vi "SA Cond - t0; Merge 2 wForms.vi"(1 "Waveform IN 2":waveform(dbl), 3 "Waveform IN 1":waveform(dbl)) -> (17 "Merged Waveform":waveform(dbl))   [LabVIEW 2022 SP3, in "GSwFormDSP.lvclass"]
uses:
  GSwFormDSP.lvclass
  Generic Utilities_class/Generic Utilities.lvclass
panel:
  out "t0 IN 1 + duration":i64
  out "t0 IN 2":i64
  out "t0 IN 1 + Duration":ext format="%.16f"
  out "t0 IN 2":ext format="%.16f"
  out "t0 IN 1":ext format="%#_24g"
  out "Duration":ext format="%#_24g"
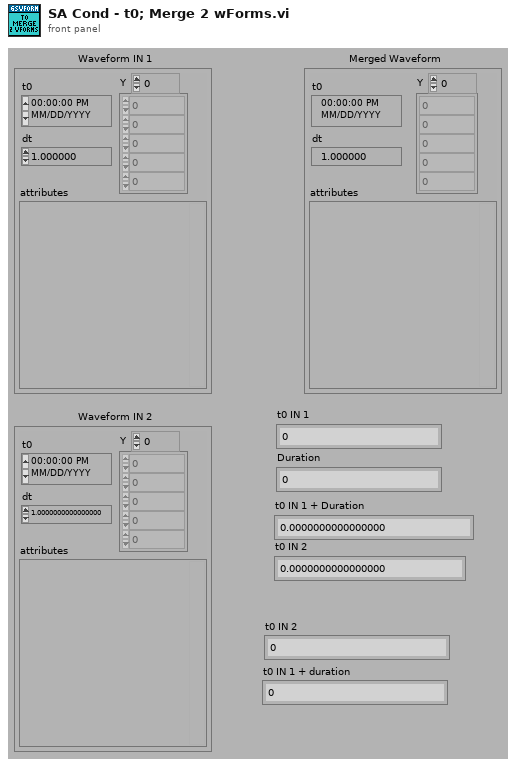
[diagram p1: front panel]
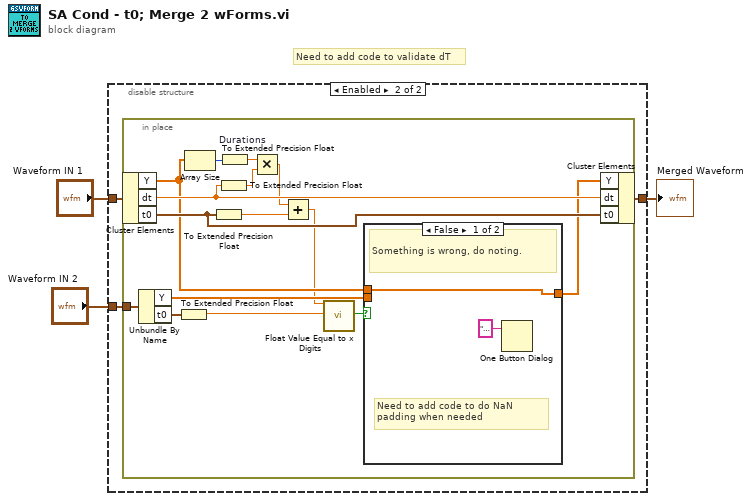
[diagram p0: block diagram]
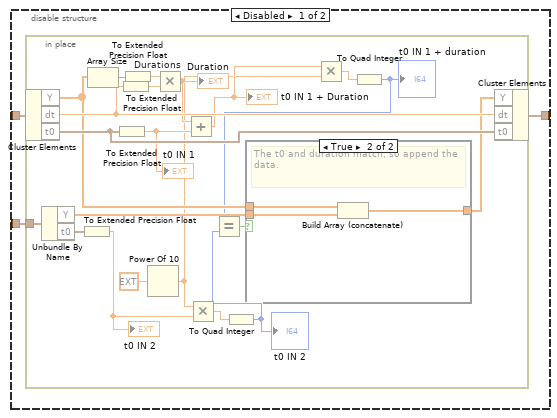
[diagram p2: hidden frame]
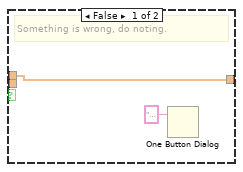
[diagram p3: hidden frame]
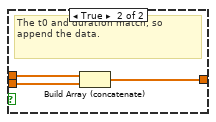
[diagram p4: hidden frame]
diagram:
  # "Need to add code to validate dT"
  n1 = disable-structure shown="Enabled" {
    disable-tunnel: "Waveform IN 1" -> [w6 w35]
    disable-tunnel: "Waveform IN 2" -> [w5 w34]
    disable-tunnel: [w4 w33] -> w1
    frame Disabled {
      n2 = in-place {
        in-place-border: w5 -> [w27]
        n3 = in-place-cluster #1(w6) -> ("Y"=w19:dbl[], "dt"=w25:dbl, "t0"=w24:timestamp)
        n4 = Unbundle By Name(w27) -> ("Y"=w18:dbl[], "t0"=w21:timestamp)
        n5 = To Extended Precision Float(1:w21) -> (0:w13:ext)
        "t0 IN 2" <- w13
        n6 = Array Size(array=w19) -> (size(s)=w22:i32)
        n7 = To Extended Precision Float(1:w24) -> (0:w16:ext)
        "t0 IN 1" <- w16
        n8 = To Extended Precision Float(1:w25) -> (0:w15:ext)
        n9 = To Extended Precision Float(1:w22) -> (0:w26:ext)
        n10 = Power Of 10(x=ext 10.0) -> (10^x=w11:ext)
        n11 = Multiply "Durations"(x=w26, y=w15) -> (x*y=w23:ext)
        "Duration" <- w23
        n12 = Add(x=w23, y=w16) -> (x+y=w12:ext)
        "t0 IN 1 + Duration" <- w12
        n13 = Multiply(x=w11, y=w13) -> (x*y=w7:ext)
        n14 = To Quad Integer(1:w7) -> (0:w10:i64)
        "t0 IN 2" <- w10
        n15 = Multiply(x=w12, y=w11) -> (x*y=w8:ext)
        n16 = To Quad Integer(1:w8) -> (0:w9:i64)
        "t0 IN 1 + duration" <- w9
        n17 = Equal?(x=w9, y=w10) -> (x = y?=w20:bool)
        n18 = case shown="True" w20 {
          tunnel: w19 -> [w29 w32]
          tunnel: w18 -> [_ w31]
          tunnel: [w29 w30] -> w17
          frame False {
            # "Something is wrong, do noting."
            n19 = One Button Dialog(message="Something wrong with t0 and waveform duration during merging of the waveforms.  The waveform will NOT be merged!!!") -> ()  [unwired: 1 in, 1 out]
          }
          frame True {
            # "The t0 and duration match, so append the data."
            n20 = Build Array (concatenate)(w32, w31) -> (w30:dbl[])
          }
        }
        n21 = in-place-cluster #1("Y"=w17, "dt"=w25, "t0"=w24) -> (w4:waveform(dbl))
      }
    }
    frame Enabled {
      n22 = in-place {
        in-place-border: w34 -> [w50]
        n23 = in-place-cluster #2(w35) -> ("Y"=w43:dbl[], "dt"=w48:dbl, "t0"=w47:timestamp)
        n24 = Unbundle By Name(w50) -> ("Y"=w42:dbl[], "t0"=w44:timestamp)
        n25 = To Extended Precision Float(1:w44) -> (0:w36:ext)
        n26 = Array Size(array=w43) -> (size(s)=w45:i32)
        n27 = To Extended Precision Float(1:w47) -> (0:w40:ext)
        n28 = To Extended Precision Float(1:w48) -> (0:w39:ext)
        n29 = To Extended Precision Float(1:w45) -> (0:w49:ext)
        n30 = Multiply "Durations"(x=w49, y=w39) -> (x*y=w46:ext)
        n31 = Add(x=w46, y=w40) -> (x+y=w37:ext)
        n32 = call "Float Value Equal to x Digits.vi"("Value A"=w37, "Value B"=w36) -> ("Equal?"=w38:bool)  [unwired: 17 in]
        n33 = case shown="False" w38 {
          tunnel: w43 -> [w52 w55]
          tunnel: w42 -> [_ w54]
          tunnel: [w52 w53] -> w41
          frame False {
            # "Need to add code to do NaN padding when needed"
            # "Something is wrong, do noting."
            n34 = One Button Dialog(message="Something wrong with t0 and waveform duration during merging of the waveforms.  The waveform will NOT be merged!!!") -> ()  [unwired: 1 in, 1 out]
          }
          frame True {
            # "The t0 and duration match, so append the data."
            n35 = Build Array (concatenate)(w55, w54) -> (w53:dbl[])
          }
        }
        n36 = in-place-cluster #2("Y"=w41, "dt"=w48, "t0"=w47) -> (w33:waveform(dbl))
      }
    }
  }
  "Merged Waveform" <- w1
